vi "Flock_Logger_Process.vi"(11 "Process":string) -> ()   [LabVIEW 2014, in "Logger.lvlib"]
doc: "This asynchronous VI is launched by the Central Process. It receives status and error messages and logs them to C:\\FlockLog.txt. It will shutdown when it recieves an exit command from the Central Process."
uses:
  Logger.lvlib
  LocalProcessMessaging/Flock_Shared_LocalProcessMessaging.lvlib
  CentralProcessMessaging/Flock_Shared_CentralProcessMessaging.lvlib
  Error Handling/Flock_ErrorHandling.lvlib
panel:
  out "Debug Status Message Value":string
  in  "error in (no error)":errorcluster
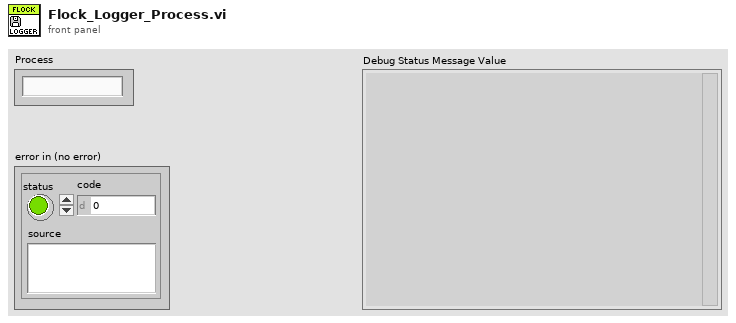
[diagram p1: front panel]
types:
  T1 = typedef "Flock_Shared_Messaging.lvlib/ProcessList.ctl" = string
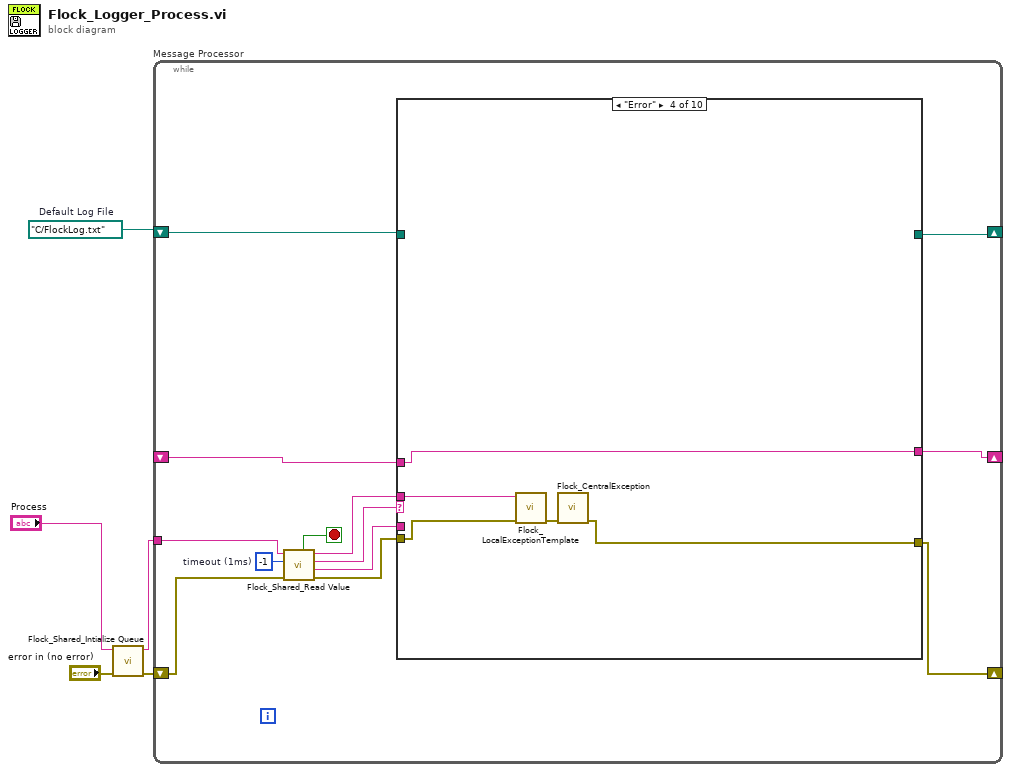
[diagram p0: block diagram]
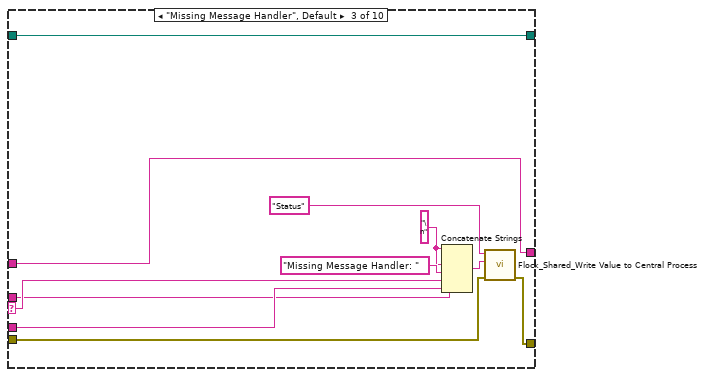
[diagram p4: hidden frame]
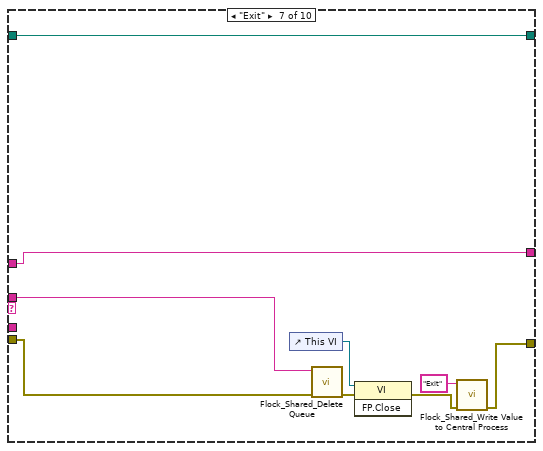
[diagram p7: hidden frame]
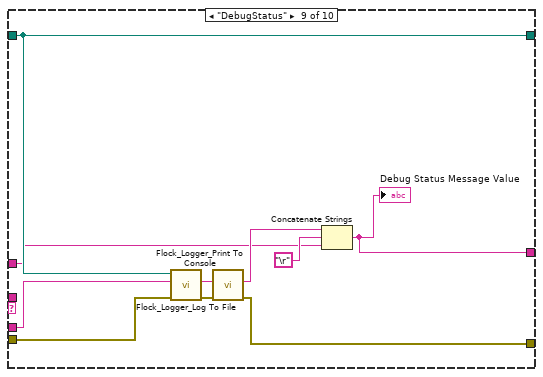
[diagram p9: hidden frame]
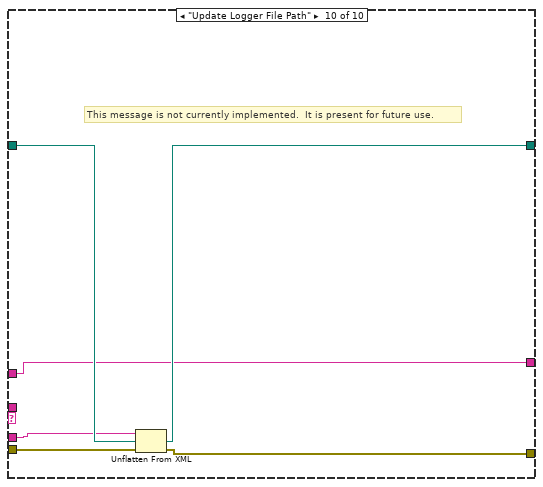
[diagram p10: hidden frame]
diagram:
  w3 = path "C:/FlockLog.txt"  # Default Log File
  n1 = call "Flock_Shared_Intialize Queue.vi"("error in (no error)"="error in (no error)", "Enum"="Process") -> ("error out"=w5:errorcluster, "Process Name"=w2:T1)  [unwired: 8 in]
  n2 = while "Message Processor" {
    shift-left: w5 -> [w18]
    shift-right: [w9] -> _
    tunnel: w2 -> [w14]
    shift-right: [w11] -> _
    shift-left: w3 -> [w12]
    shift-right: [w6] -> _
    shift-left: _ -> [w7]
    stop <- w8 stop-if-true
    w15 = -1  # timeout (1ms)
    n3 = call "Flock_Shared_Read Value.vi"("error in (no error)"=w18, "timeout (1ms)"=w15, "Process"=w14) -> ("error out"=w16:errorcluster, "Message Value"=w13:string, "Message Name"=w17:string, "Process"=w10:T1, "Exit Process"=w8:bool)  [unwired: 4 in]
    n4 = case shown="\"Error\"" w17 {
      selector: w17 -> [_ _ w27 _ _ _ _ _ _ _]
      tunnel: w16 -> [w20 w23 w33 w38 w41 w44 w49 w55 w64 w69]
      tunnel: [w20 w23 w32 w37 w41 w44 w46 w55 w62 w67] -> w9
      tunnel: w13 -> [_ _ w26 _ _ _ _ _ w61 w70]
      tunnel: w12 -> [_ w22 w31 _ _ w43 w52 _ w65 w71]
      tunnel: [_ w22 w31 _ _ w43 w52 _ w65 w68] -> w11
      tunnel: w10 -> [_ _ w25 w36 _ _ w53 _ _ _]
      tunnel: w7 -> [w19 w21 w24 w35 w40 w42 w50 w54 w57 w66]
      tunnel: [w19 w21 w24 w35 w40 w42 w50 w54 w56 w66] -> w6
      frame "---------- Framework Operations ----------" {
        # "Dummy case to add a seperator in the Case Structure menu"
      }
      frame "", "Idle" {
      }
      frame "Missing Message Handler", Default {
        w29 = "\n" ("string")
        n5 = Concatenate Strings(w29, w25, w29, "Missing Message Handler: " ("string"), w27, w26) -> (w28:string)
        n6 = call "Flock_Shared_Write Value to Central Process.vi"("error in (no error)"=w33, "Message Value"=w28, "Message Name"="Status") -> ("error out"=w32:errorcluster)  [unwired: 8 in]
      }
      frame "Error" {
        n7 = call "Flock_LocalExceptionTemplate.vi"("Error In"=w38, "Process List"=w36) -> ("Error Out"=w39:errorcluster)  [unwired: 9 in]
        n8 = call "Flock_CentralException.vi"("Error In"=w39) -> ("Error Out"=w37:errorcluster)  [unwired: 10 in]
      }
      frame "---------- Generic Operations ----------" {
        # "Dummy case to add a seperator in the Case Structure menu"
      }
      frame "Initialize" {
      }
      frame "Exit" {
        n9 = control-ref of="This VI"() -> (w51:refnum<vi>)
        n10 = call "Flock_Shared_Delete Queue.vi"("Error In"=w49, "Process Name"=w53) -> ("Error Out"=w48:errorcluster)  [unwired: 9 in]
        n11 = invoke class="VI" method="FP.Close"(reference=w51, error in=w48) -> (error out=w47:errorcluster)  [unwired: 1 in, 2 out]
        n12 = call "Flock_Shared_Write Value to Central Process.vi"("error in (no error)"=w47, "Message Name"="Exit") -> ("error out"=w46:errorcluster)  [unwired: 9 in]
      }
      frame "---------- Application Operations ----------" {
      }
      frame "DebugStatus" {
        n13 = call "Flock_Logger_Log To File.vi"("error in"=w64, "Text"=w61, "File"=w65) -> ("error out"=w63:errorcluster, "TextOut"=w60:string)  [unwired: 7 in]
        n14 = call "Flock_Logger_Print To Console.vi"("Error In"=w63, "Text"=w60) -> ("Error Out"=w62:errorcluster, "TextOut"=w59:string)  [unwired: 8 in]
        n15 = Concatenate Strings(w59, "\r", w57) -> (w56:string)
        "Debug Status Message Value" <- w56
      }
      frame "Update Logger File Path" {
        # "This message is not currently implemented.  It is present for future use."
        n16 = Unflatten From XML(xml string=w70, type=w71, error in (no error)=w69) -> (value=w68:path, error out=w67:errorcluster)
      }
    }
  }
